vi "Camera_angle.vi"() -> ()   [LabVIEW 2019]
panel:
  in  "Camera a":dbl
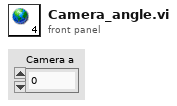
[diagram p1: front panel]
diagram:
